vi "HRTF-Set Multiplexer (TDT).vi"(0 "iAzimuth":i32, 5 "MUX 1":i32, 7 "MUX 2":i32, 11 "error in (no error)":errorcluster) -> (15 "error out":errorcluster)   [LabVIEW 2020]
uses:
  PXI DAQ VIs/TDT VIs/TDT-Globals.vi
panel:
  out "WordOut":u8[](array[numeric]) format="%08b"
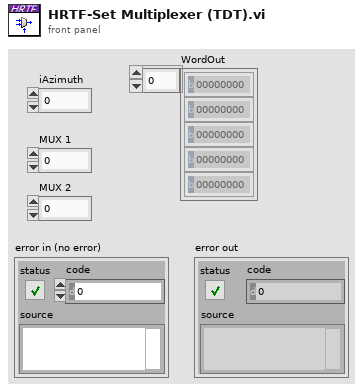
[diagram p1: front panel]
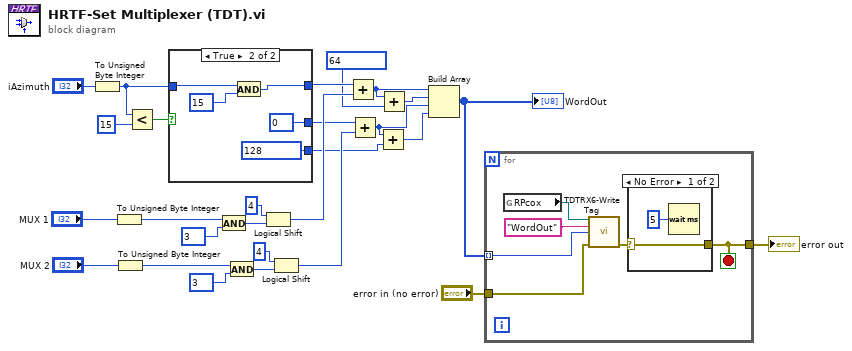
[diagram p0: block diagram]
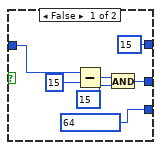
[diagram p3: hidden frame]
diagram:
  n1 = To Unsigned Byte Integer(number="iAzimuth") -> (unsigned 8bit integer=w24:u8)
  n2 = To Unsigned Byte Integer(number="MUX 1") -> (unsigned 8bit integer=w18:u8)
  n3 = To Unsigned Byte Integer(number="MUX 2") -> (unsigned 8bit integer=w14:u8)
  n4 = Less?(x=w24, y=u8 15) -> (x < y?=w26:bool)
  n5 = case shown="True" w26 {
    tunnel: w24 -> [w33 w39]
    tunnel: [u8 15 ("y") w37] -> w13
    tunnel: [w29 u8 0 ("y")] -> w11
    tunnel: [u8 64 ("y") u8 128 ("y")] -> w3
    frame False {
      n6 = Subtract(x=w33, y=u8 15) -> (x-y=w30:u8)
      n7 = And(x=w30, y=u8 15) -> (x .and. y?=w29:u8)
    }
    frame True {
      n8 = And(x=w39, y=u8 15) -> (x .and. y?=w37:u8)
    }
  }
  n9 = And(x=w18, y=u8 3) -> (x .and. y?=w20:u8)
  n10 = And(x=w14, y=u8 3) -> (x .and. y?=w16:u8)
  n11 = Logical Shift(y=i16 4, x=w20) -> (x << y=w12:u8)
  n12 = Logical Shift(y=i16 4, x=w16) -> (x << y=w10:u8)
  n13 = Add(x=w13, y=w12) -> (x+y=w5:u8)
  n14 = Add(x=w11, y=w10) -> (x+y=w4:u8)
  n15 = Add(x=w4, y=w3) -> (x+y=w2:u8)
  n16 = Add(x=w5, y=u8 64) -> (x+y=w7:u8)
  n17 = Build Array(w5, w7, w4, w2) -> (w9:u8[])
  "WordOut" <- w9
  n18 = for {
    tunnel: w9 -> [w44] mode=indexing
    tunnel: "error in (no error)" -> [w43]
    tunnel: [w41] -> w1
    stop <- w41 stop-if-true
    n19 = global read "TDT-Globals.vi" "RPcox"() -> (w40:refnum<k7>)
    n20 = call "TDTRX6-Write Tag.vi"("RPcox"=w40, "Name"="WordOut", "Value"=w44, "error in"=w43) -> ("error out"=w42:errorcluster)  [unwired: 10 in, 1 out]
    n21 = case shown="No Error" w42 {
      selector: w42 -> [w47 w48]
      tunnel: [w47 w48] -> w41
      frame No Error {
        n22 = Wait (ms)(milliseconds to wait=u32 5) -> ()  [unwired: 1 out]
      }
      frame Error {
      }
    }
  }
  "error out" <- w1
